vi "TW Substitute the assigned name for lib and lvclass.vi"(8 "error in":errorcluster, 10 "Project Name":string, 11 "Name to Lib Map":map{string, refnum<vi>}(c390)) -> (0 "error out":errorcluster, 3 "Name to Lib Map out":map{string, refnum<vi>}(c390))   [LabVIEW 2021, in "Plugin Generator.lvlib"]
uses:
  Plugin Generator.lvlib
  <vilib>/Utility/EditLVLibs/Edit LVLibs.lvlib
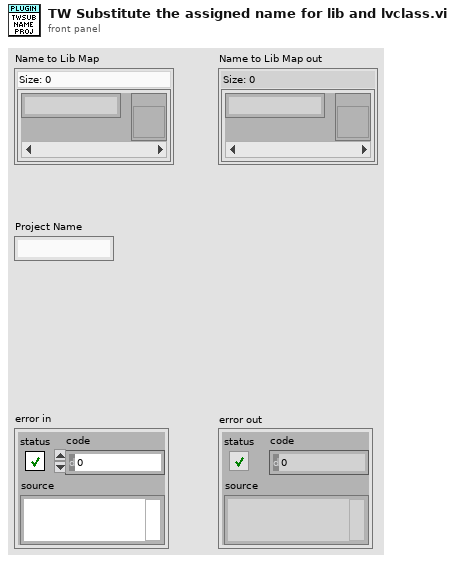
[diagram p1: front panel]
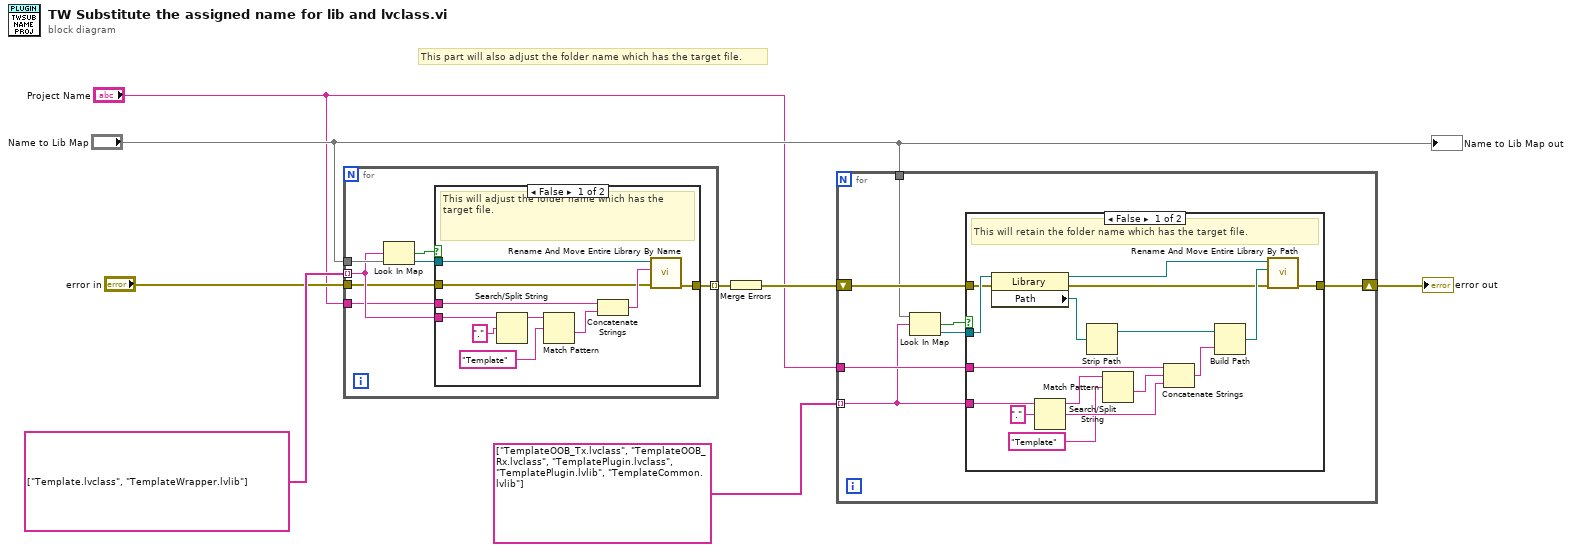
[diagram p0: block diagram]
diagram:
  # "This part will also adjust the folder name which has the target file."
  n1 = for {
    tunnel: string[] ["Template.lvclass", "TemplateWrapper.lvlib"] -> [w13] mode=indexing
    tunnel: "Name to Lib Map" -> [w15]
    tunnel: [w12] -> w3 mode=indexing
    tunnel: "Project Name" -> [w10]
    tunnel: "error in" -> [w9]
    n2 = Look In Map(map=w15, key=w13) -> (key not found?=w14:bool, value=w11:refnum<vi>)  [unwired: 1 in]
    n3 = case shown="False" w14 {
      tunnel: w13 -> [w24 _]
      tunnel: [w21 w26] -> w12
      tunnel: w11 -> [w19 _]
      tunnel: w10 -> [w18 _]
      tunnel: w9 -> [w17 w26]
      frame False {
        # "This will adjust the folder name which has the target file."
        n4 = Search/Split String(string=w24, search string/char (-)=".") -> (substring before match=w22:string)  [unwired: 1 in, 2 out]
        n5 = Match Pattern(string=w22, regular expression="Template") -> (after substring=w16:string)  [unwired: 1 in, 3 out]
        n6 = Concatenate Strings(w18, w16) -> (w20:string)
        n7 = call <vilib>:"Rename And Move Entire Library By Name.vi"("error in (no error)"=w17, "New name without file extension"=w20, "Library ref in"=w19) -> ("error out"=w21:errorcluster)  [unwired: 6 in, 2 out]
      }
      frame True {
      }
    }
  }
  n8 = Merge Errors(w3) -> (w7:errorcluster)
  n9 = for {
    tunnel: "Name to Lib Map" -> [w29]
    tunnel: "Project Name" -> [w28]
    shift-right: [w31] -> w8
    shift-left: w7 -> [w30]
    tunnel: string[] ["TemplateOOB_Tx.lvclass", "TemplateOOB_Rx.lvclass", "TemplatePlugin.lvclass", "TemplatePlugin.lvlib", "TemplateCommon.lvlib"] -> [w27] mode=indexing
    n10 = Look In Map(map=w29, key=w27) -> (key not found?=w32:bool, value=w33:refnum<vi>)  [unwired: 1 in]
    n11 = case shown="False" w32 {
      tunnel: w33 -> [w39 _]
      tunnel: w27 -> [w47 _]
      tunnel: [w40 w50] -> w31
      tunnel: w28 -> [w38 _]
      tunnel: w30 -> [w37 w50]
      frame False {
        # "This will retain the folder name which has the target file."
        n12 = property class="Library"(reference=w39, error in=w37) -> (reference out=w42:refnum<vi>, error out=w36:errorcluster, "Path"=w49:path)
        n13 = Search/Split String(string=w47, search string/char (-)=".") -> (substring before match=w45:string, match + rest of string=w43:string)  [unwired: 1 in, 1 out]
        n14 = Strip Path(path=w49) -> (stripped path=w48:path)  [unwired: 1 out]
        n15 = Match Pattern(string=w45, regular expression="Template") -> (after substring=w34:string)  [unwired: 1 in, 3 out]
        n16 = Concatenate Strings(w38, w34, w43) -> (w44:string)
        n17 = Build Path(base path=w48, name or relative path=w44) -> (appended path=w41:path)
        n18 = call <vilib>:"Rename And Move Entire Library By Path.vi"("error in (no error)"=w36, "New library path"=w41, "Library ref in"=w42) -> ("error out"=w40:errorcluster)  [unwired: 7 in, 1 out]
      }
      frame True {
      }
    }
  }
  "error out" <- w8
  "Name to Lib Map out" <- "Name to Lib Map"
